vi "dataCommon.vi"(8 "error in (no error)":errorcluster, 11 "Command Text":string) -> (0 "error out":errorcluster, 3 "Data":string[][](array[string]))   [LabVIEW 2014]
uses:
  <vilib>/addons/database/Connection.llb/DB Tools Open Connec (String).vi
  <vilib>/addons/database/Connection.llb/Conn Execute.vi
  <vilib>/addons/database/Recordset.llb/Rec Fetch Recordset Data (R).vi
  <vilib>/addons/database/Recordset.llb/Rec Destroy - Connection.vi
  <vilib>/addons/database/_DB Variant To Data/Database Variant To Data.xnode
  <vilib>/addons/database/NI_Database_API.lvlib
panel:
  in  "error in (no error) 3":errorcluster
  out "error out 3":errorcluster
  in  "SQL query":string
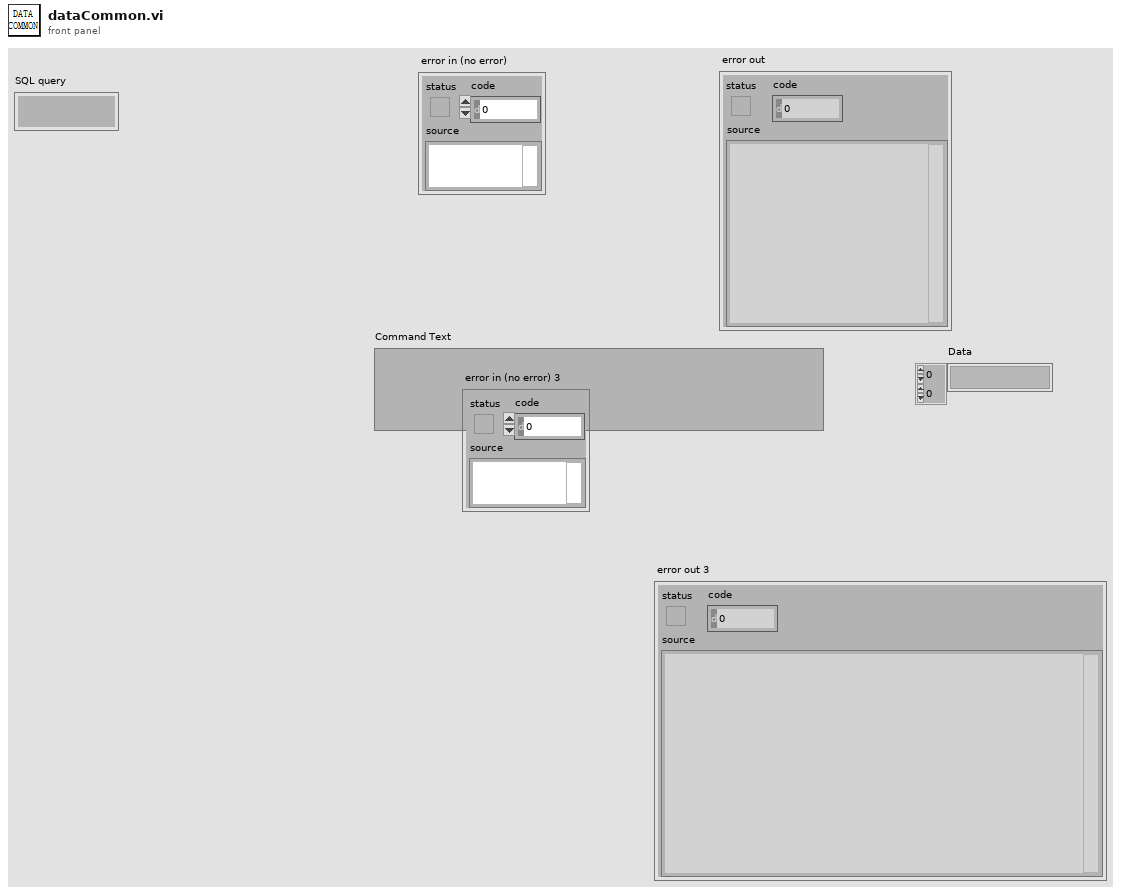
[diagram p1: front panel]
types:
  T1 = enum32{"invalid app kind", "Development System", "Run Time System", "Student Edition", "Embedded LabVIEW", "Evaluation", "Custom"}
  T2 = typedef "NI_Database_API.lvlib/Conn ObjectReference.ctl" = refnum<k1>
  T3 = typedef "NI_Database_API.lvlib/Rec ObjectReference.ctl" = refnum<k1>
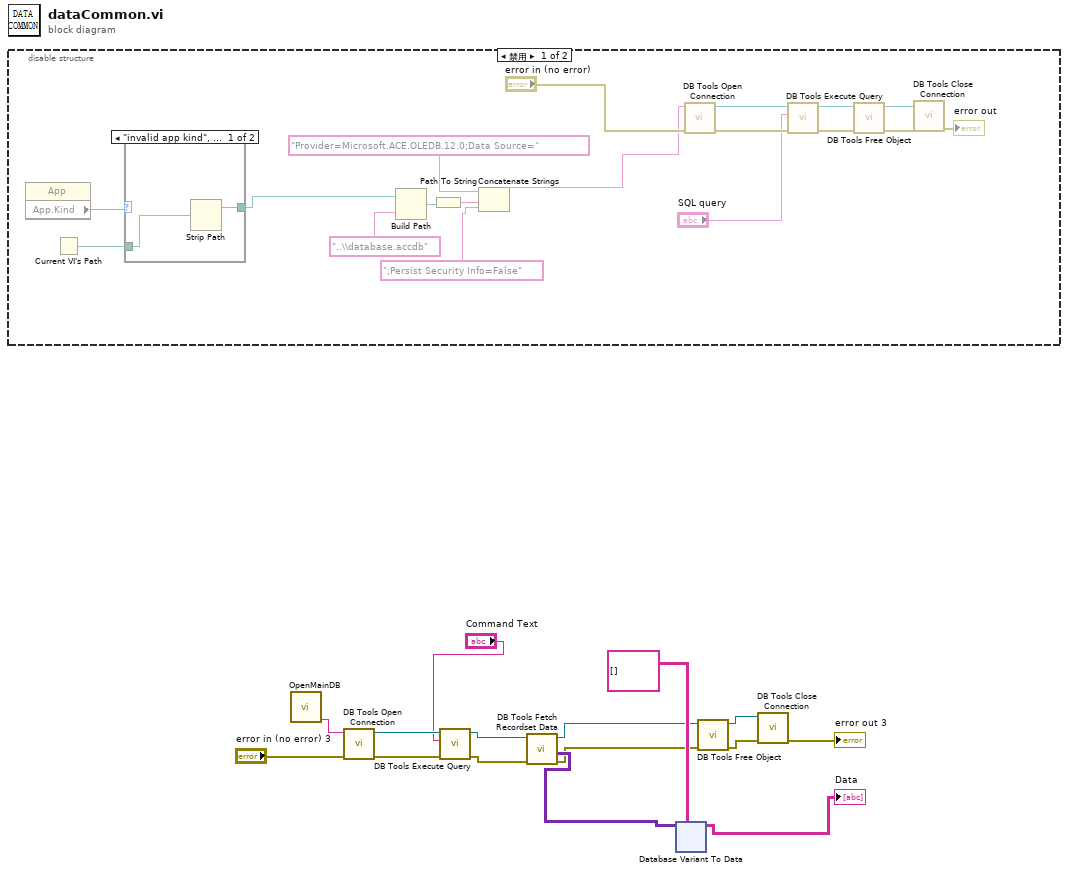
[diagram p0: block diagram]
diagram:
  n1 = disable-structure shown="禁用" {
    frame Disabled {
      n2 = property class="App"() -> ("App.Kind"=w17:T1)  [unwired: 2 in, 2 out]
      n3 = Current VI's Path() -> (path=w18:path)
      n4 = case shown="\"invalid app kind\", 默认" w17 {
        tunnel: w18 -> [w35 w36]
        tunnel: [w34 w36] -> w19
        frame "invalid app kind", Default {
          n5 = Strip Path(path=w35) -> (stripped path=w34:path)  [unwired: 1 out]
        }
        frame "Development System" {
        }
      }
      n6 = Build Path(base path=w19, name or relative path="..\\database.accdb" ("名称或相对路径")) -> (appended path=w21:path)
      n7 = Path To String(path=w21) -> (string=w22:string)
      n8 = Concatenate Strings("Provider=Microsoft.ACE.OLEDB.12.0;Data Source=", w22, ";Persist Security Info=False") -> (w31:string)
      n9 = call-poly <vilib>:"DB Tools Open Connection.vi"("error in (no error)"="error in (no error)", "connection information"=w31) -> ("error out"=w29:errorcluster, "connection reference"=w30:T2)  [unwired: 6 in]
      n10 = call-poly <vilib>:"DB Tools Execute Query.vi"("error in (no error)"=w29, "SQL query"="SQL query", "connection reference"=w30) -> ("error out"=w27:errorcluster, "recordset reference"=w28:T3)  [unwired: 5 in]
      n11 = call-poly <vilib>:"DB Tools Free Object.vi"("error in (no error)"=w27, "recordset reference"=w28) -> ("error out"=w25:errorcluster, "connection reference"=w26:T2)  [unwired: 8 in]
      n12 = call <vilib>:"DB Tools Close Connection.vi"("error in (no error)"=w25, "connection reference"=w26) -> ("error out"=→"error out":errorcluster)  [unwired: 5 in]
    }
    frame Enabled {
    }
  }
  n13 = call "OpenMainDB.vi"() -> ("头信息"=w3:string)  [unwired: 11 in]
  n14 = call-poly <vilib>:"DB Tools Open Connection.vi"("error in (no error)"="error in (no error) 3", "connection information"=w3) -> ("error out"=w7:errorcluster, "connection reference"=w6:T2)  [unwired: 6 in]
  n15 = call-poly <vilib>:"DB Tools Execute Query.vi"("error in (no error)"=w7, "SQL query"="Command Text", "connection reference"=w6) -> ("error out"=w8:errorcluster, "recordset reference"=w5:T3)  [unwired: 5 in]
  n16 = call-poly <vilib>:"DB Tools Fetch Recordset Data.vi"("error in (no error)"=w8, "recordset reference"=w5) -> ("error out"=w10:errorcluster, "recordset data"=w15:variant[][], "recordset reference out"=w9:T3)  [unwired: 3 in]
  n17 = xnode "Database Variant To Data"("database variant"=w15, "type"=string[][] []) -> ("data"=→"Data":string[][])  [unwired: 1 in, 1 out]
  n18 = call-poly <vilib>:"DB Tools Free Object.vi"("error in (no error)"=w10, "recordset reference"=w9) -> ("error out"=w12:errorcluster, "connection reference"=w11:T2)  [unwired: 8 in]
  n19 = call <vilib>:"DB Tools Close Connection.vi"("error in (no error)"=w12, "connection reference"=w11) -> ("error out"=→"error out 3":errorcluster)  [unwired: 5 in]
